vi "obtainObservableList.vi"(5 "ExplodeContainer (F)":bool, 7 "AllHierarchy (T)":bool=TRUE, 8 "error in":errorcluster, 9 "ObservableData":variant, 10 "ObservableName":string) -> (0 "error out":errorcluster, 1 "ObservableValue":variant[](array[variant]), 2 "ObservableName":string[](array[string]))   [LabVIEW 2025, in "ObserverClass.lvlib"]
uses:
  ObserverClass.lvlib
  <vilib>/Utility/Data Type/Type Definitions/Data Type.ctl
  <vilib>/Utility/Data Type/NI_Data Type.lvlib
  <vilib>/PNR/LabVIEW Composition/Composition/Composition.lvlib
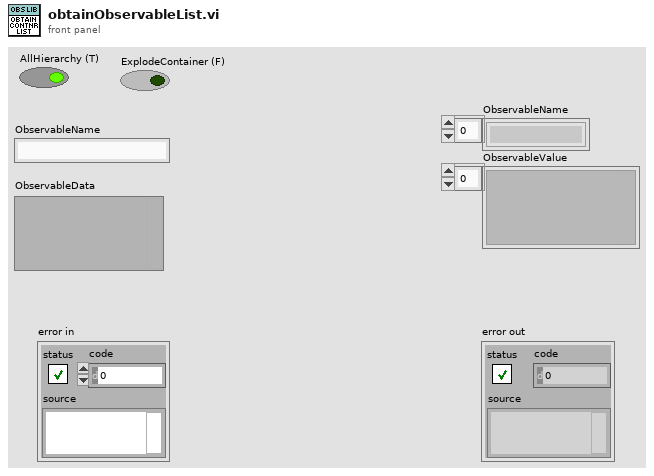
[diagram p1: front panel]
types:
  T1 = typedef "NI_Data Type.lvlib/Data Type.ctl" = enum8{"Invalid Type", "Void", "I8", "I16", "I32", "I64", "U8", "U16", "U32", "U64", "Single Float", "Double Float", "Extended Float", "Single Complex", "Double Complex", "Extended Complex", "Enum U8", "Enum U16", "Enum U32", "Enum U64", "Single Float With Unit", "Double Float With Unit", "Extended Float With Unit", "Single Complex with Unit", "Double Complex with Unit", "Extended Complex with Unit", "Boolean", "String", "Path", "Picture", "Tag", "Array", "Cluster", "Variant", "LV Variant", "Waveform", "Timestamp", "Digital Waveform", "Digital Data", "ExpressData", "Refnum", "External Data", "VI", "Poly VI", "LabVIEW Class Instance", "Fixed Point", "Set Collection", "Map Collection"}
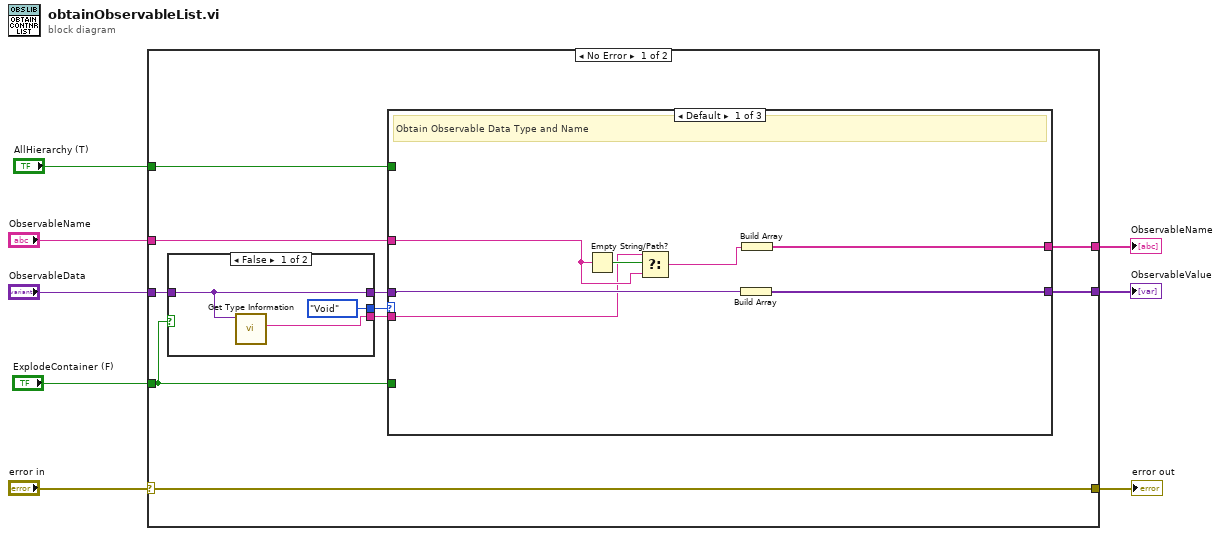
[diagram p0: block diagram]
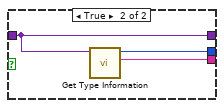
[diagram p2: hidden frame]
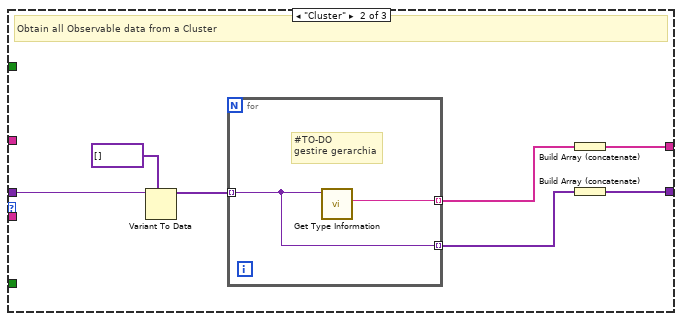
[diagram p3: hidden frame]
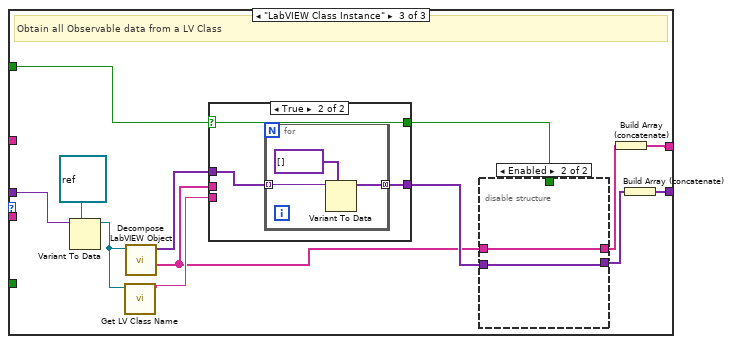
[diagram p4: hidden frame]
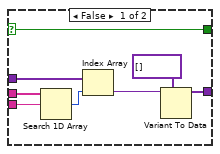
[diagram p6: hidden frame]
diagram:
  n1 = case shown="No Error" "error in" {
    selector: "error in" -> [w18 w77]
    tunnel: [w18 w77] -> w7
    tunnel: [w17 _] -> w4
    tunnel: [w16 _] -> w3
    tunnel: "ObservableData" -> [w15 _]
    tunnel: "AllHierarchy (T)" -> [w12 _]
    tunnel: "ObservableName" -> [w11 _]
    tunnel: "ExplodeContainer (F)" -> [w10 _]
    frame No Error {
      n2 = case shown="False" w10 {
        tunnel: w15 -> [w20 w22]
        tunnel: [Data_Type."Void" ("type") w24] -> w14
        tunnel: [w19 w23] -> w13
        tunnel: [w20 w22] -> w9
        frame False {
          n3 = call <vilib>:"Get Type Information.vi"("variant"=w20) -> ("name"=w19:string)  [unwired: 6 in, 4 out]
        }
        frame True {
          n4 = call <vilib>:"Get Type Information.vi"("variant"=w22) -> ("name"=w23:string, "type"=w24:T1)  [unwired: 6 in, 3 out]
        }
      }
      n5 = case shown="Default" w14 {
        tunnel: [w29 w38 w42] -> w17
        tunnel: [w30 w37 w43] -> w16
        tunnel: w9 -> [w31 w36 w45]
        tunnel: w13 -> [w25 _ _]
        tunnel: w12 -> [_ _ w41]
        tunnel: w11 -> [w27 _ _]
        tunnel: w10 -> [_ _ _]
        frame Default {
          # "Obtain Observable Data Type and Name"
          n6 = Empty String/Path?(string/path=w27) -> (empty?=w28:bool)
          n7 = Select(t=w25, s=w28, f=w27) -> (s? t:f=w26:string)
          n8 = Build Array(w31) -> (w30:variant[])
          n9 = Build Array(w26) -> (w29:string[])
        }
        frame "Cluster" {
          # "Obtain all Observable data from a Cluster"
          n10 = Variant To Data(type=variant[] [], Variant=w36) -> (data=w34:variant[])  [unwired: 1 in, 1 out]
          n11 = for {
            tunnel: w34 -> [w39] mode=indexing
            tunnel: [w40] -> w33 mode=indexing
            tunnel: [w39] -> w32 mode=indexing
            # "#TO-DO\ngestire gerarchia"
            n12 = call <vilib>:"Get Type Information.vi"("variant"=w39) -> ("name"=w40:string)  [unwired: 6 in, 4 out]
          }
          n13 = Build Array (concatenate)(w33) -> (w38:string[])
          n14 = Build Array (concatenate)(w32) -> (w37:variant[])
        }
        frame "LabVIEW Class Instance" {
          # "Obtain all Observable data from a LV Class"
          n15 = Variant To Data(type=refnum<class> refnum ("LabVIEW Object"), Variant=w45) -> (data=w49:refnum<class>)  [unwired: 1 in, 1 out]
          n16 = call <vilib>:"Get LV Class Name.vi"("object"=w49) -> ("class name"=w48:string)  [unwired: 9 in, 1 out]
          n17 = call <vilib>:"Decompose LabVIEW Object.vi"("LabVIEW Object"=w49) -> ("Class Names"=w44:string[], "Private Data Clusters"=w47:variant[])  [unwired: 7 in, 2 out]
          n18 = case shown="True" w41 {
            selector: w41 -> [w63 w71]
            tunnel: w47 -> [w68 w73]
            tunnel: [w70 w72] -> w52
            tunnel: w44 -> [w66 _]
            tunnel: w48 -> [w65 _]
            tunnel: [w63 w71] -> w46
            frame False {
              n19 = Search 1D Array(1D array=w66, element=w65) -> (index of element=w67:i32)  [unwired: 1 in]
              n20 = Index Array(array=w68, index=w67) -> (element=w69:variant)
              n21 = Variant To Data(type=variant[] [], Variant=w69) -> (data=w70:variant[])  [unwired: 1 in, 1 out]
            }
            frame True {
              n22 = for {
                tunnel: w73 -> [w75] mode=indexing
                tunnel: [w74] -> w72 mode=concatenating
                n23 = Variant To Data(type=variant[] [], Variant=w75) -> (data=w74:variant[])  [unwired: 1 in, 1 out]
              }
            }
          }
          n24 = disable-structure shown="Enabled" {
            disable-tunnel: w52 -> [w58 w61]
            disable-tunnel: [w57 w61] -> w51
            disable-tunnel: [w56 w62] -> w50
            disable-tunnel: w46 -> [w55 _]
            disable-tunnel: w44 -> [w54 w62]
            frame Disabled {
              n25 = for {
                tunnel: w58 -> [w60] mode=indexing
                tunnel: [w59] -> w56 mode=concatenating
                tunnel: [w60] -> w57 mode=concatenating
                tunnel: w55 -> [_]
                tunnel: w54 -> [w59] mode=indexing
              }
            }
            frame Enabled {
            }
          }
          n26 = Build Array (concatenate)(w50) -> (w42:string[])
          n27 = Build Array (concatenate)(w51) -> (w43:variant[])
        }
      }
    }
    frame Error {
    }
  }
  "error out" <- w7
  "ObservableName" <- w4
  "ObservableValue" <- w3
